vi "ForebrainArbiter.vi"(0 "WaypointInput":dbl[](array[numeric]), 5 "Beh2Input":dbl[](array[numeric]), 7 "HypoInput":dbl[](array[numeric]), 11 "Beh3Input":dbl[](array[numeric])) -> (6 "ForebrainActCom":dbl[](array[numeric]))   [LabVIEW 2010]
doc: "This VI arbitrates command input from theNeo-Cortex, and Hypothallumus THINK processes and conducts a voting poll arbitor with input from each to determine the one output command.\n\nInputs: 90 cell arrays of weighted direction commands \n\nOutput: Cluster of desried velocity and direction"
panel:
  out "Waveform Graph":dbl[][](graph)
  # "This subVI takes the four\nBehavior commands; three from the Neo-Cortex \nand one from theHypoThallumus and\naverages them"
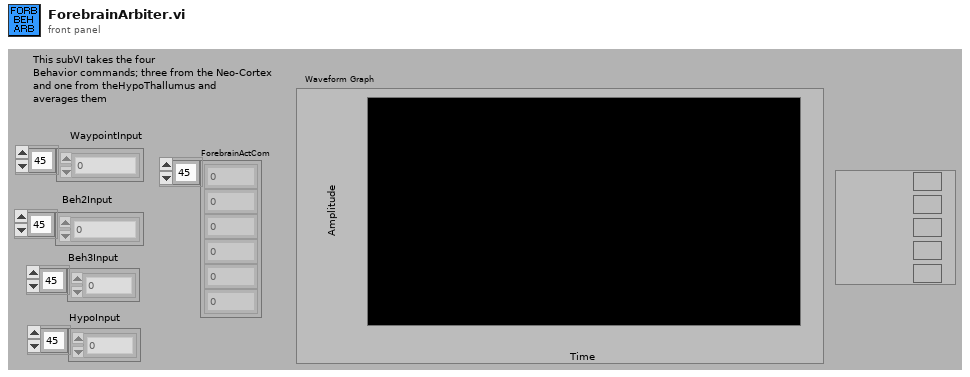
[diagram p1: front panel]
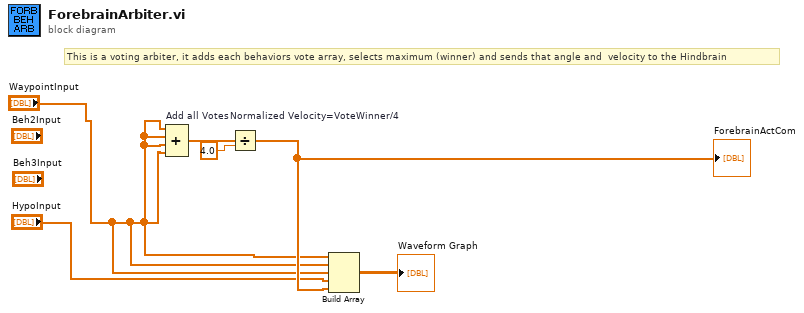
[diagram p0: block diagram]
diagram:
  # "This is a voting arbiter, it adds each behaviors vote array, selects maximum (winner) and sends that angle and  velocity to the Hindbrain"
  n1 = Compound Arithmetic op=ADD "Add all Votes"("WaypointInput", "WaypointInput", "WaypointInput", "WaypointInput") -> (w5:dbl[])
  n2 = Divide "Normalized Velocity=VoteWinner/4"(x=w5, y=4.0) -> (x/y=w3:dbl[])
  "ForebrainActCom" <- w3
  n3 = Build Array "Build Array"("WaypointInput", "WaypointInput", "WaypointInput", "HypoInput", w3) -> (→"Waveform Graph":dbl[][])
